vi "Komponetnen und Gasnummer in LIN Polynom setzen.vi"(8 "Fehler (Eingang, kein Fehler)":errorcluster, 10 "Komponentenauswahl":T1(array[cluster]), 11 "Gasnummer":T2 min=1 max=5) -> (0 "Fehler (Ausgang)":errorcluster, 2 "Lin-Polynom":T3 {"zusätzliche Zeitdauer Erster Punkt" format="%#_5g"; "Lin Modus" items=["Cal Gas to PNS", "Cal Gas to Samplepoint", "Measure"]; "Gas Ablaufdatum" format="%<%d.%m.%Y>T"; "HovaCAL Flow AutoLin"."HovaCAL Flow Input Cluster" format="%.2f"; "Gasflasche" items=["----"=10000, "IAG MG"=0, "IAG NH3 3000"=1, "IAG NH3 2000"=2, "IAG NH3 200"=3]; "Conditions:" items=["field", "laboratory"]; "Kalibrierauswahl" items=["Inaktiv", "Aktiv"]; "Anzahl Stufen" format="%#_5g"; "Zeitdauer Stufe" format="%#_5g"; "Verdünnungsgas" items=["N2", "O2"]; "Komponentenauswahl"."Konzentration" format="%#.6f"; "Gasnummer:" min=1 max=5; "Prüfgas Konzentration" format="%#.6f"; "Polynomkoeff." format="%#_18f"}, 3 "Gasnummer out":T2 min=1 max=5)   [LabVIEW 2020, in "Linearisierung v2.lvlib" / "SpanEinstellungen.lvlib"]
uses:
  SpanEinstellungen.lvlib
  Lin-Polynom Daten.ctl
  KomponentenArray.ctl
  Visualisierungs Elemente/Auswahlfeld.ctl
  Visualisierungs Elemente/Zahlen-Eingabefeld.ctl
  EPA Optionsfeld.ctl
  Gasteiler/HovaCal/AutoLin Hovacal.ctl
  Kalibrieroption.ctl
  EPA1065-307/Condition.ctl
  Seiten/System Einstellungen V2/Konfig Gasflasche.ctl
  Seiten/System Einstellungen V2/Gasflasche Auswahl.ctl
  Gasteiler/HovaCAL_Interface/Controls/Flow Einstellung.ctl
  Gasteiler/HovaCAL_Interface/Controls/Pump state.ctl
  Seiten/CalGas Aufschaltung/Lin Modus.ctl
  Gasnumber.ctl
  Aktion Lin Daten aufarbeiten.ctl
  Linearisierung v2.lvlib
  Gasteiler/Gasteiler.lvlib
  Gasteiler/HovaCal/HovaCal.lvlib
  EPA1065-307/Linearity verification 1065-307.lvlib
  Seiten/System Einstellungen V2/System Einstellungen V2.lvlib
  Gasteiler/HovaCAL_Interface/Controls/Controls.lvlib
  Seiten/CalGas Aufschaltung/CalGas Aufschaltung.lvlib
panel:
  # "%"
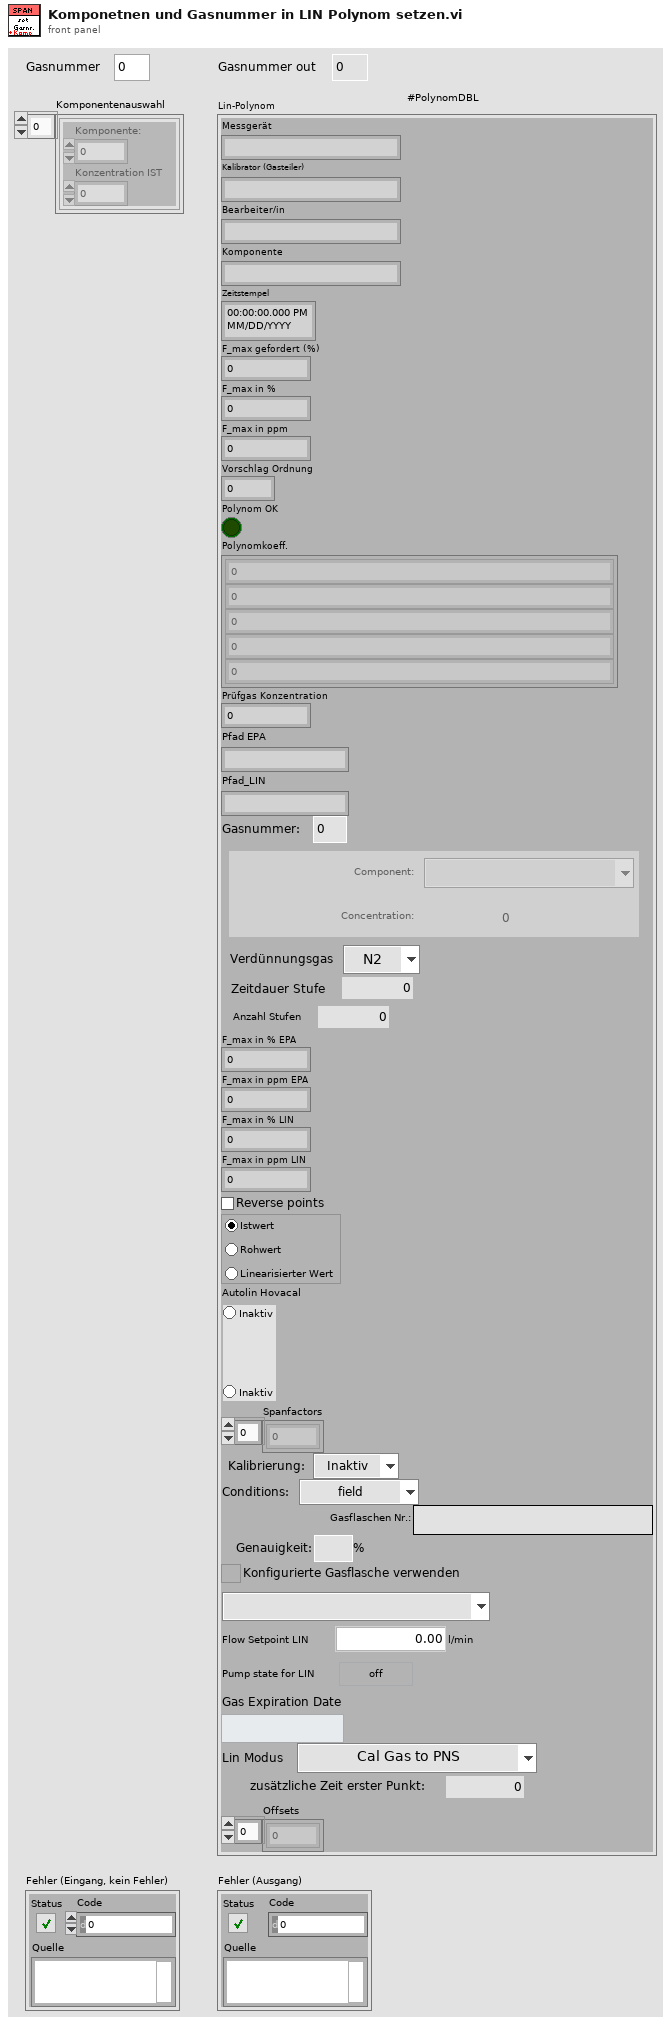
[diagram p1: front panel]
types:
  T1 = cluster{"Komponente:":u16, "Konzentration IST":dbl}[]
  T2 = typedef "Linearisierung v2.lvlib/Gasnumber.ctl" = u8
  T3 = typedef "Linearisierung v2.lvlib/Lin-Polynom Daten.ctl" = cluster{"Messgerät":string, "Kalibrator (Gasteiler)":string, "Bearbeiter/in":string, "Komponente":string, "Zeitstempel":timestamp, "F_max gefordert (%)":sgl, "F_max in %":sgl, "F_max in ppm":sgl, "Vorschlag Ordnung":i32, "Polynom OK":bool, "Polynomkoeff.":dbl[], "Prüfgas Konzentration":dbl, "Pfad EPA":string, "Pfad_LIN":string, "Gasnummer:":u8, "Komponentenauswahl":T4, "Verdünnungsgas":T6, "Zeitdauer Stufe":T7, "Anzahl Stufen":T7, "F_max in % EPA":sgl, "F_max in ppm EPA":sgl, "F_max in % LIN":sgl, "F_max in ppm LIN":sgl, "Punkte umkehren":bool, "EPA Optionsfeld":T8, "Autolin Hovacal":T9, "Spanfactors":sgl[], "Kalibrierauswahl":T10, "Conditions:":T11, "Gasflaschen Nr.:":string, "Bottle Accuracy":dbl, "Konfig Gasflasche":T12, "Gasflasche":T13, "HovaCAL Flow AutoLin":T14, "MFC Output":T15, "Gas Ablaufdatum":timestamp, "Lin Modus":T16, "zusätzliche Zeitdauer Erster Punkt":sgl, "Offsets":sgl[]}
  T4 = typedef "Linearisierung v2.lvlib/KomponentenArray.ctl" = cluster{"Komponente:":T5, "Konzentration":dbl}[]
  T5 = typedef "Auswahlfeld.ctl" = u16
  T6 = typedef "Linearisierung v2.lvlib/Gasteiler.lvlib/Prüfgas in.ctl" = u16
  T7 = typedef "Zahlen-Eingabefeld.ctl" = sgl
  T8 = typedef "Linearisierung v2.lvlib/EPA Optionsfeld.ctl" = enum32{"Istwert", "Rohwert", "Linearisierter Wert"}
  T9 = typedef "Linearisierung v2.lvlib/Gasteiler.lvlib/HovaCal.lvlib/AutoLin Hovacal.ctl" = enum32{"Keine Auswahl", "Optionsauswahl 1", "Optionsauswahl 2"}
  T10 = typedef "Linearisierung v2.lvlib/Kalibrieroption.ctl" = u16
  T11 = typedef "Linearisierung v2.lvlib/Linearity verification 1065-307.lvlib/Condition.ctl" = u16
  T12 = typedef "System Einstellungen V2.lvlib/Konfig Gasflasche.ctl" = bool
  T13 = typedef "System Einstellungen V2.lvlib/Gasflasche Auswahl.ctl" = u16
  T14 = typedef "Linearisierung v2.lvlib/Gasteiler.lvlib/HovaCAL_Interface.lvlib/Controls.lvlib/Flow Einstellung.ctl" = cluster{"HovaCAL Flow Input Cluster":dbl}
  T15 = typedef "Linearisierung v2.lvlib/Gasteiler.lvlib/HovaCAL_Interface.lvlib/Controls.lvlib/Pump state.ctl" = cluster{"Run":bool}
  T16 = typedef "CalGas Aufschaltung.lvlib/Lin Modus.ctl" = u16
  T17 = typedef "Linearisierung v2.lvlib/Aktion Lin Daten aufarbeiten.ctl" = enum16{"lesen", "Protkolldaten", "speichern", "laden", "EPA auswerten", "Tabelle schreiben", "Lin auswerten", "Tab init", "Stufentabelle", "EPA aktiviert", "Nachbehandlung laden", "Tabelle löschen", "Istwerte löschen", "Zeile löschen", "Zeile einfügen", "LIN aktiviert", "LIN/EPA aktiv laden", "EGAK Tab", "LIN übernehmen", "Tab init ohne Stufen"}
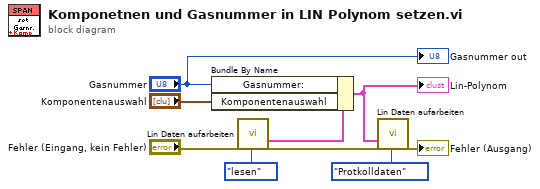
[diagram p0: block diagram]
diagram:
  n1 = call "Lin Daten aufarbeiten.vi"("error in (no error)"="Fehler (Eingang, kein Fehler)", "Aktionen"=Aktion_Lin_Daten_aufarbeiten."lesen") -> ("Lin-Polynom"=w6:T3, "error out"=w4:errorcluster)  [unwired: 15 in, 9 out]
  n2 = Bundle By Name(cluster=w6, "Gasnummer:"="Gasnummer", "Komponentenauswahl"="Komponentenauswahl") -> (w3:T3)
  "Lin-Polynom" <- w3
  n3 = call "Lin Daten aufarbeiten.vi"("Lin-Polynom"=w3, "error in (no error)"=w4, "Aktionen"=Aktion_Lin_Daten_aufarbeiten."Protkolldaten") -> ("error out"=→"Fehler (Ausgang)":errorcluster)  [unwired: 14 in, 10 out]
  "Gasnummer out" <- "Gasnummer"
